vi "ParseXML.vi"(8 "error in (no error)":errorcluster, 11 "Node":refnum<k20>) -> (0 "error out":errorcluster)   [LabVIEW 2017]
uses:
  <resource>/objmgr/DOMUserDefRef.rc
panel:
  out "Node Name":string
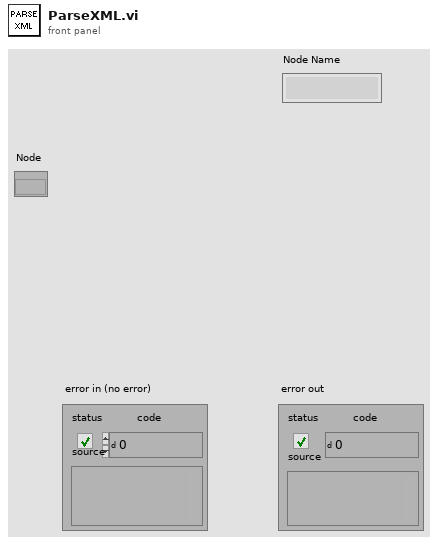
[diagram p1: front panel]
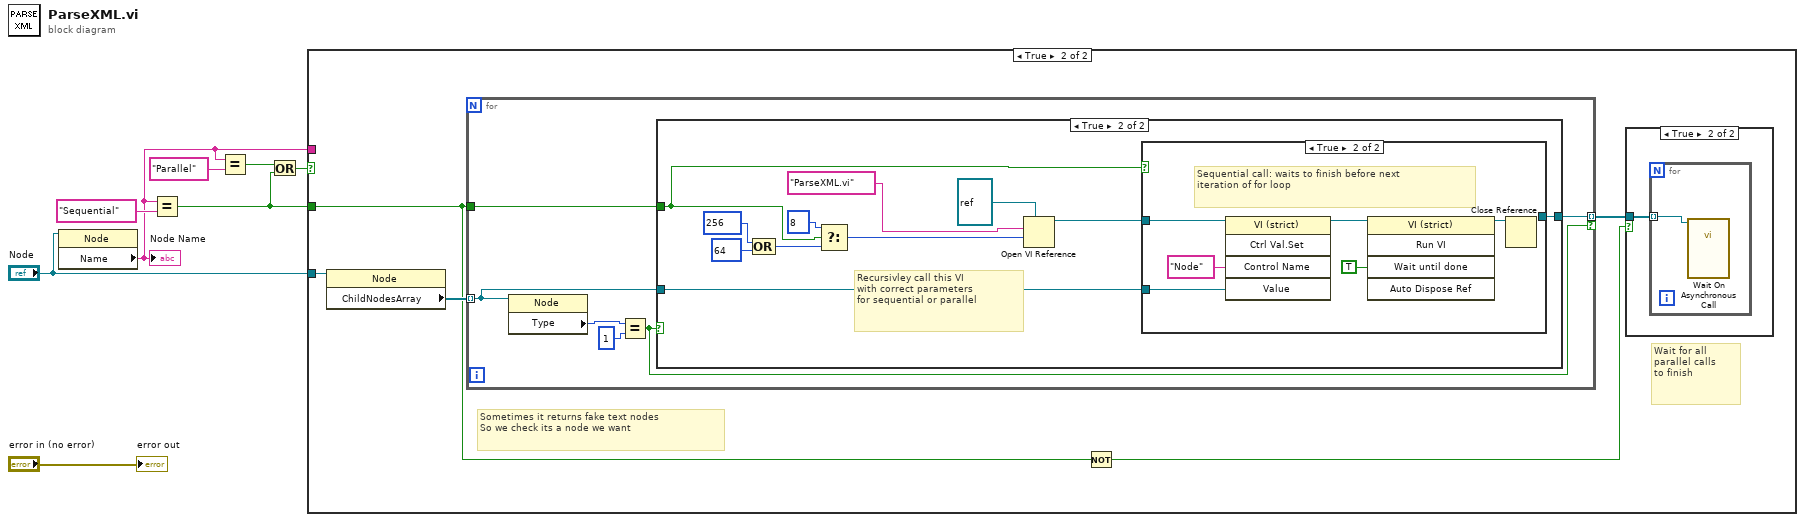
[diagram p0: block diagram]
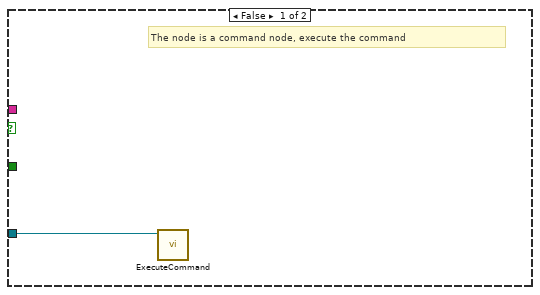
[diagram p2: hidden frame]
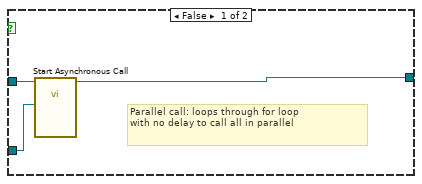
[diagram p5: hidden frame]
diagram:
  n1 = property class="Node"(reference="Node") -> ("Name"=w2:string)  [unwired: 1 in, 2 out]
  "Node Name" <- w2
  n2 = Equal?(x=w2, y="Sequential") -> (x = y?=w3:bool)
  n3 = Equal?(x=w2, y="Parallel") -> (x = y?=w5:bool)
  n4 = Or(x=w5, y=w3) -> (x .or. y?=w4:bool)
  n5 = case shown="True" w4 {
    tunnel: "Node" -> [w9 w13]
    tunnel: w3 -> [_ w10]
    tunnel: w2 -> [_ _]
    frame False {
      # "The node is a command node, execute the command"
      n6 = call "ExecuteCommand.vi"("Node"=w9) -> ()  [unwired: 11 in]
    }
    frame True {
      # "Wait for all\nparallel calls\nto finish"
      # "Sometimes it returns fake text nodes\nSo we check its a node we want"
      n7 = property class="Node"(reference=w13) -> ("ChildNodesArray"=w14:refnum<k20>[])  [unwired: 1 in, 2 out]
      n8 = for {
        tunnel: w14 -> [w20] mode=indexing
        tunnel: w10 -> [w18]
        tunnel: [w19] -> w12 mode=indexing if=w17
        n9 = property class="Node"(reference=w20) -> ("Type"=w21:i32)  [unwired: 1 in, 2 out]
        n10 = Equal?(x=w21, y=1) -> (x = y?=w17:bool)
        n11 = case shown="True" w17 {
          tunnel: w18 -> [_ w33]
          tunnel: w20 -> [_ w29]
          tunnel: [_ w23] -> w19
          frame False {
          }
          frame True {
            # "Recursivley call this VI\nwith correct parameters\nfor sequential or parallel"
            n12 = Compound Arithmetic op=OR(256 ("options"), 64 ("options")) -> (w32:i32)
            n13 = Select(t=8 ("options"), s=w33, f=w32) -> (s? t:f=w31:i32)
            n14 = Open VI Reference(type specifier VI Refnum (for type only)=refnum<vi> refnum ("VI Refnum"), vi path="ParseXML.vi" ("name or relative path"), options=w31) -> (vi reference=w25:refnum<vi>)  [unwired: 3 in, 1 out]
            n15 = case shown="True" w33 {
              tunnel: w29 -> [w35 w42]
              tunnel: w25 -> [w36 w37]
              tunnel: [w34 _] -> w23
              frame False {
                # "Parallel call: loops through for loop\nwith no delay to call all in parallel"
                n16 = call-by-ref "Start Asynchronous Call"(reference=w36, "Node"=w35) -> (reference out=w34:refnum<vi>)  [unwired: 11 in, 2 out]
              }
              frame True {
                # "Sequential call: waits to finish before next\niteration of for loop"
                n17 = invoke class="VI (strict)" method="Ctrl Val.Set"(reference=w37, "Control Name"="Node", "Value"=w42) -> (reference out=w40:refnum<vi>)  [unwired: 2 in, 4 out]
                n18 = invoke class="VI (strict)" method="Run VI"(reference=w40, "Wait until done"=TRUE ("Wait Until Done")) -> (reference out=w38:refnum<vi>)  [unwired: 3 in, 4 out]
                n19 = Close Reference(reference=w38) -> ()  [unwired: 1 in, 1 out]
              }
            }
          }
        }
      }
      n20 = Not(x=w10) -> (.not. x?=w11:bool)
      n21 = case shown="True" w11 {
        tunnel: w12 -> [_ w15]
        frame False {
        }
        frame True {
          n22 = for {
            tunnel: w15 -> [w16] mode=indexing
            n23 = call-by-ref "Wait On Asynchronous Call"(reference=w16) -> ()  [unwired: 12 in, 3 out]
          }
        }
      }
    }
  }
  "error out" <- "error in (no error)"
